vi "Camera Communication.vi"(9 "Modle":string="1", 10 "Trigger Cammand":bool) -> ()   [LabVIEW 2015]
uses:
  Control Button/cameraenum.ctl
  Galobal variable_TI.vi
panel:
  out "error out 2":errorcluster
  out "Boolean":bool
  in  "x":bool
  out "data out 3":string
  out "data out 2":string
  out "error out":errorcluster
  out "data out":string
  # "Meadium=1"
  # "Globle=2"
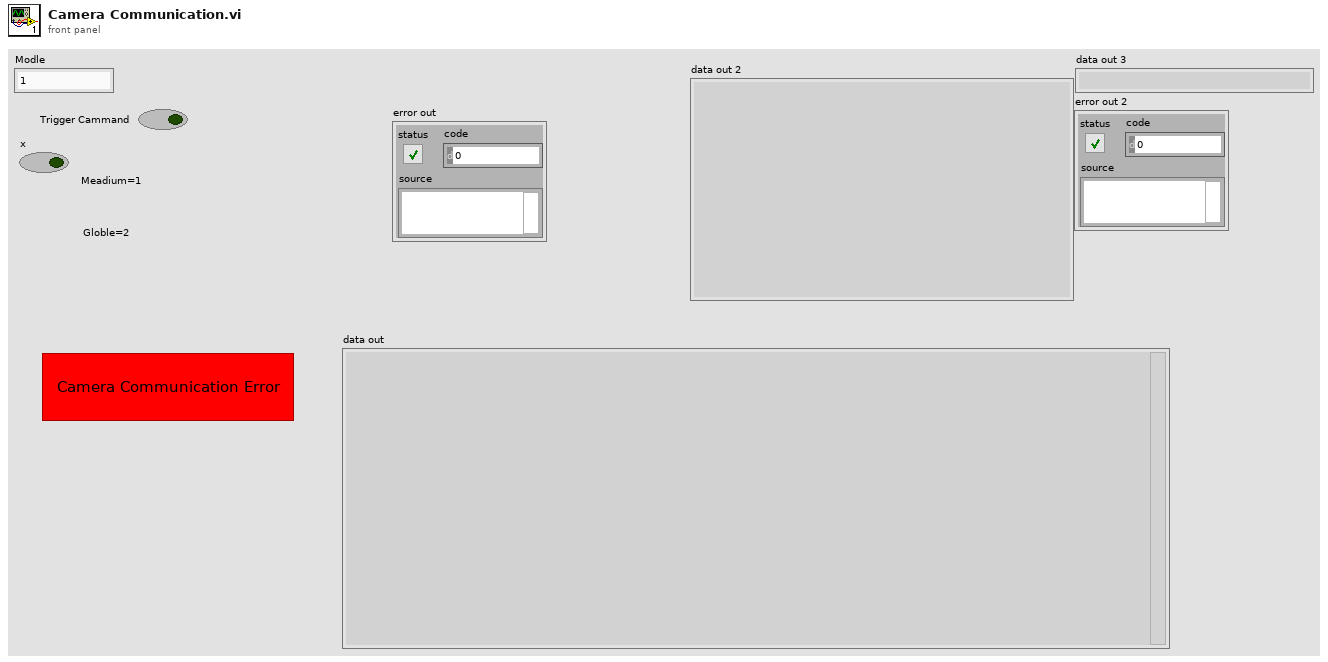
[diagram p1: front panel]
types:
  T1 = enum16{"Standard", "Buffered", "CRLF", "Immediate"}
  T2 = typedef "cameraenum.ctl" = enum16{"Poll event", "Camera Off Mode", "Job Chage", "Camera online  Mode", "Camera trigger Mode", "Read", "Session close"}
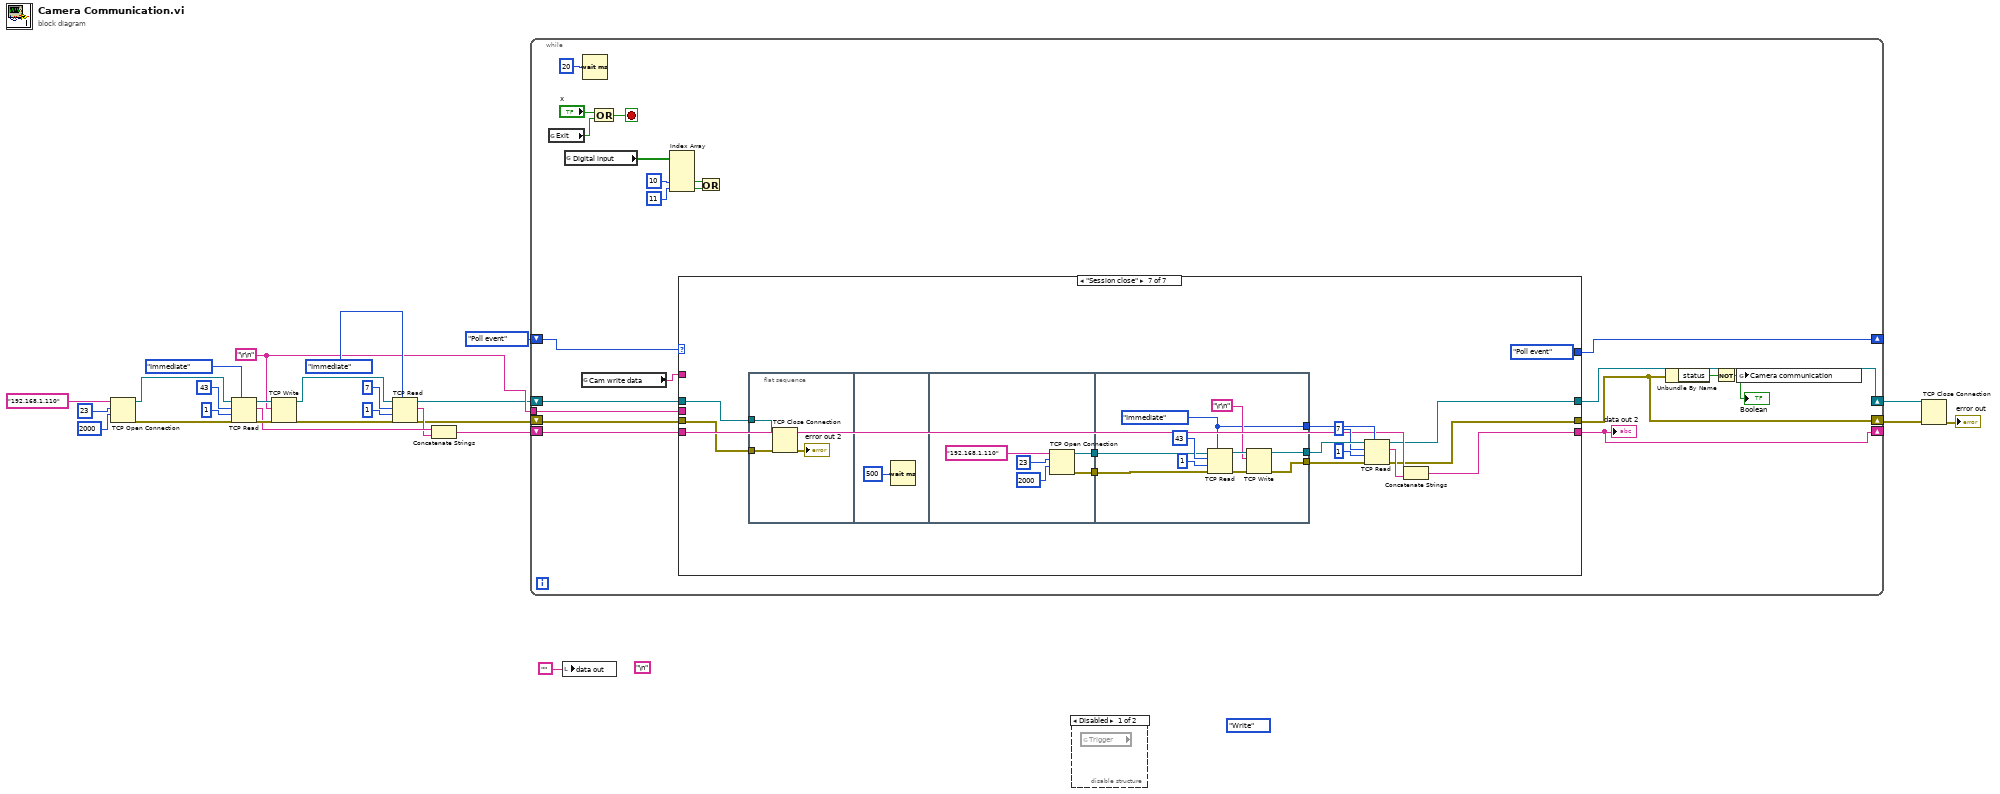
[diagram p0: block diagram]
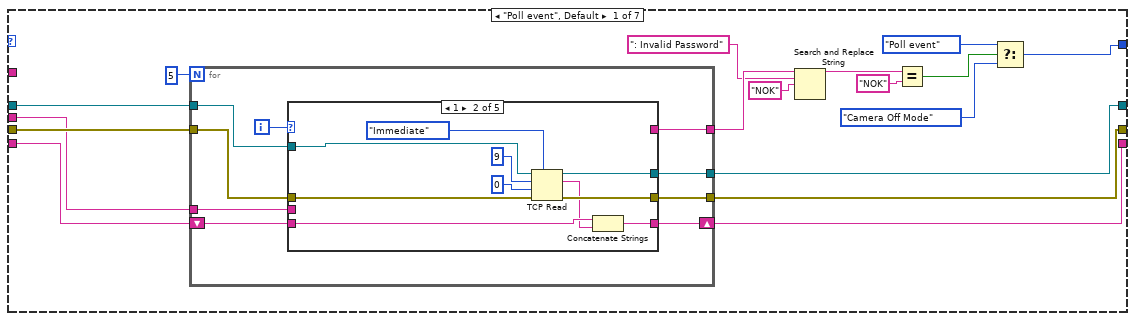
[diagram p3: hidden frame]
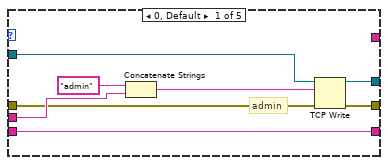
[diagram p4: hidden frame]
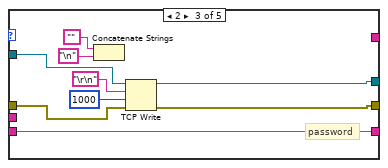
[diagram p5: hidden frame]
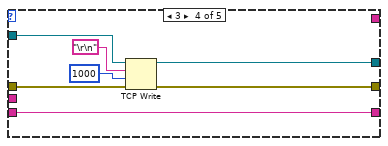
[diagram p6: hidden frame]
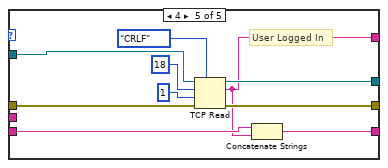
[diagram p7: hidden frame]
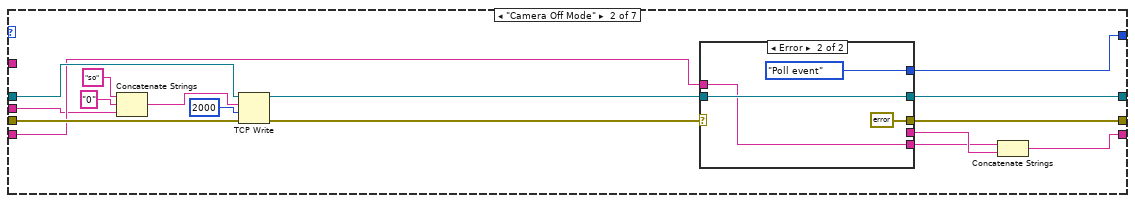
[diagram p8: hidden frame]
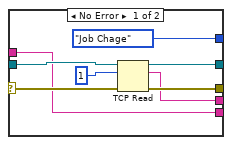
[diagram p9: hidden frame]
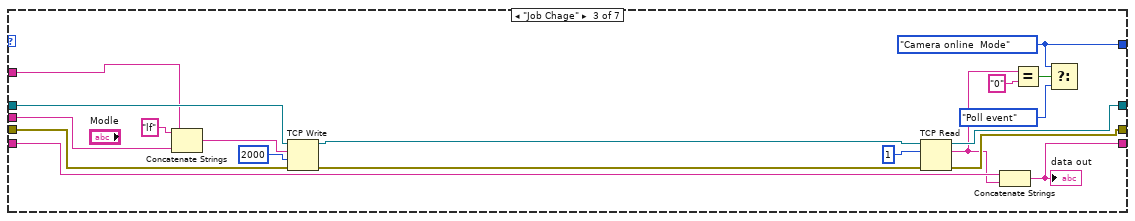
[diagram p10: hidden frame]
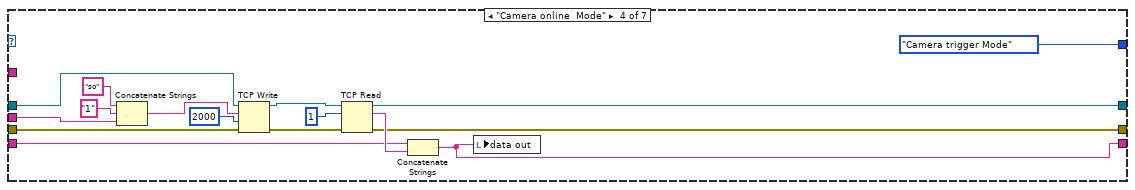
[diagram p11: hidden frame]
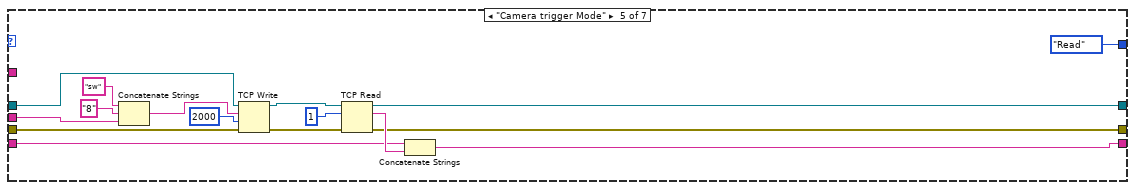
[diagram p12: hidden frame]
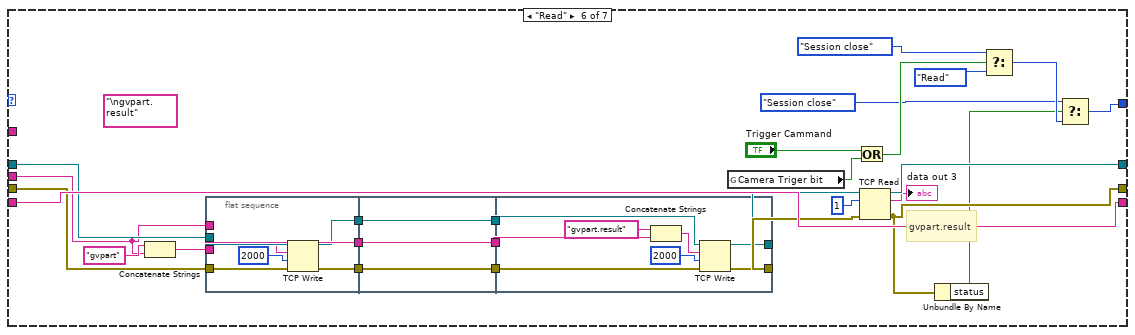
[diagram p13: hidden frame]
diagram:
  (unwired) "\n"
  w4 = "\r\n"
  (unwired) enum16{"Poll event", "Write", "Read", ""}."Write"
  n1 = TCP Open Connection(address="192.168.1.110", remote port or service name=u16 23, timeout ms (60000)=2000) -> (connection ID=w20:refnum<k5>, error out=w19:errorcluster)  [unwired: 2 in]
  n2 = TCP Read(connection ID=w20, bytes to read=43, error in (no error)=w19, 7:T1."Immediate" ("mode (standard)"), 9:1 ("timeout ms (25000)")) -> (connection ID out=w18:refnum<k5>, data out=w15:string, error out=w17:errorcluster)
  n3 = TCP Write(connection ID=w18, data in=w4, error in (no error)=w17) -> (connection ID out=w13:refnum<k5>, error out=w12:errorcluster)  [unwired: 1 in, 1 out]
  n4 = TCP Read(connection ID=w13, bytes to read=7, error in (no error)=w12, 7:T1."Immediate" ("mode (standard)"), 9:1 ("timeout ms (25000)")) -> (connection ID out=w2:refnum<k5>, data out=w14:string, error out=w1:errorcluster)
  n5 = Concatenate Strings(w15, w14) -> (w3:string)
  n6 = while {
    shift-right: [w46] -> _
    shift-left: w3 -> [w45]
    shift-right: [w43] -> _
    shift-left: cameraenum."Poll event" ("Enum") -> [w42]
    shift-right: [w32] -> w6
    shift-left: w2 -> [w47]
    shift-right: [w31] -> w5
    shift-left: w1 -> [w30]
    tunnel: w4 -> [w41]
    stop <- w39 stop-if-true
    n7 = global read "Galobal variable_TI.vi" "Exit"() -> (w40:bool)
    n8 = global read "Galobal variable_TI.vi" "Digital input"() -> (w37:bool[])
    n9 = global read "Galobal variable_TI.vi" "Cam write data"() -> (w27:string)
    n10 = Wait (ms)(milliseconds to wait=u32 20) -> ()  [unwired: 1 out]
    n11 = Compound Arithmetic op=OR("x", w40) -> (w39:bool)
    n12 = Index Array(array=w37, index #3=10 ("index"), index #4=11 ("index")) -> (element #3=w34:bool, element #4=w33:bool)  [unwired: 2 in, 2 out]
    n13 = case shown="\"Session close\"" w42 {
      tunnel: w47 -> [w63 w133 w161 w172 w188 w218 w244]
      tunnel: w30 -> [w62 w132 w160 w171 w187 w216 w243]
      tunnel: [w60 w123 w156 w170 w186 w217 w246] -> w32
      tunnel: [w59 w127 w155 w169 w185 w203 w247] -> w31
      tunnel: [w52 w126 w147 cameraenum."Camera trigger Mode" ("Enum") cameraenum."Read" ("f") w222 cameraenum."Poll event" ("f")] -> w43
      tunnel: [w58 w120 w153 w167 w184 w223 w248] -> w46
      tunnel: w45 -> [w64 w122 w154 w168 w183 w223 w249]
      tunnel: w41 -> [w61 w121 w152 w165 w181 w207 _]
      tunnel: w27 -> [_ _ w146 _ _ _ _]
      frame "Poll event", Default {
        n14 = for {
          N: 5 -> [_]
          tunnel: w61 -> [w72]
          tunnel: w63 -> [w71]
          tunnel: w62 -> [w70]
          tunnel: [w69] -> w60
          tunnel: [w68] -> w59
          shift-right: [w67] -> w58
          shift-left: w64 -> [w66]
          tunnel: [w65] -> w51
          i -> [w73]
          n15 = case shown="1" w73 {
            tunnel: w72 -> [w80 _ _ _ _]
            tunnel: w71 -> [w78 w91 w100 w104 w116]
            tunnel: w70 -> [w77 w90 w99 w103 w108]
            tunnel: [w76 w87 w98 w107 w115] -> w69
            tunnel: [w75 w86 w97 w106 w114] -> w68
            tunnel: [w74 w89 w96 w105 w112] -> w67
            tunnel: w66 -> [w74 w88 w96 w105 w113]
            tunnel: [_ _ _ _ w111] -> w65
            frame 0, Default {
              # "admin"
              n16 = Concatenate Strings("admin", w80) -> (w79:string)
              n17 = TCP Write(connection ID=w78, data in=w79, error in (no error)=w77) -> (connection ID out=w76:refnum<k5>, error out=w75:errorcluster)  [unwired: 1 in, 1 out]
            }
            frame 1 {
              n18 = TCP Read(connection ID=w91, bytes to read=9, error in (no error)=w90, 7:T1."Immediate" ("mode (standard)"), 9:0 ("timeout ms (25000)")) -> (connection ID out=w87:refnum<k5>, data out=w84:string, error out=w86:errorcluster)
              n19 = Concatenate Strings(w88, w84) -> (w89:string)
            }
            frame 2 {
              # "password"
              n20 = Concatenate Strings("", "\n") -> ()  [unwired: 1 out]
              n21 = TCP Write(connection ID=w100, data in="\r\n", error in (no error)=w99, 9:1000 ("timeout ms (25000)")) -> (connection ID out=w98:refnum<k5>, error out=w97:errorcluster)  [unwired: 1 out]
            }
            frame 3 {
              n22 = TCP Write(connection ID=w104, data in="\r\n", error in (no error)=w103, 9:1000 ("timeout ms (25000)")) -> (connection ID out=w107:refnum<k5>, error out=w106:errorcluster)  [unwired: 1 out]
            }
            frame 4 {
              # "User Logged In"
              n23 = TCP Read(connection ID=w116, bytes to read=18, error in (no error)=w108, 7:T1."CRLF" ("mode (standard)"), 9:1 ("timeout ms (25000)")) -> (connection ID out=w115:refnum<k5>, data out=w111:string, error out=w114:errorcluster)
              n24 = Concatenate Strings(w113, w111) -> (w112:string)
            }
          }
        }
        n25 = Search and Replace String(input string=w51, search string=": Invalid Password", replace string="NOK" ("replace string (\"\")")) -> (result string=w48:string)  [unwired: 5 in, 3 out]
        n26 = Equal?(x=w48, y="NOK") -> (x = y?=w55:bool)
        n27 = Select(t=cameraenum."Poll event" ("Enum"), s=w55, f=cameraenum."Camera Off Mode") -> (s? t:f=w52:T2)
      }
      frame "Camera Off Mode" {
        n28 = Concatenate Strings("so" ("data in"), "0" ("string"), w121) -> (w129:string)
        n29 = TCP Write(connection ID=w133, data in=w129, error in (no error)=w132, 9:2000 ("timeout ms (25000)")) -> (connection ID out=w124:refnum<k5>, error out=w128:errorcluster)  [unwired: 1 out]
        n30 = case shown="Error" w128 {
          selector: w128 -> [w137 _]
          tunnel: [w136 errorcluster {"status"=FALSE, "code"=0, "source"=""} ("error IO")] -> w127
          tunnel: [cameraenum."Job Chage" ("Enum") cameraenum."Poll event" ("Enum")] -> w126
          tunnel: w124 -> [w139 w143]
          tunnel: [w138 w143] -> w123
          tunnel: w122 -> [w135 w142]
          tunnel: [w135 w142] -> w118
          tunnel: [w134 _] -> w119
          frame No Error {
            n31 = TCP Read(connection ID=w139, bytes to read=1, error in (no error)=w137) -> (connection ID out=w138:refnum<k5>, data out=w134:string, error out=w136:errorcluster)  [unwired: 2 in]
          }
          frame Error {
          }
        }
        n32 = Concatenate Strings(w118, w119) -> (w120:string)
      }
      frame "Job Chage" {
        w147 = cameraenum."Camera online  Mode" ("Enum")
        n33 = Concatenate Strings("lf" ("data in"), w146, w152) -> (w163:string)
        n34 = TCP Write(connection ID=w161, data in=w163, error in (no error)=w160, 9:2000 ("timeout ms (25000)")) -> (connection ID out=w157:refnum<k5>, error out=w159:errorcluster)  [unwired: 1 out]
        n35 = TCP Read(connection ID=w157, bytes to read=1, error in (no error)=w159) -> (connection ID out=w156:refnum<k5>, data out=w151:string, error out=w155:errorcluster)  [unwired: 2 in]
        n36 = Concatenate Strings(w154, w151) -> (w153:string)
        "data out" <- w153
        n37 = Equal?(x=w151, y="0") -> (x = y?=w149:bool)
        n38 = Select(t=w147, s=w149, f=cameraenum."Poll event" ("Enum")) -> ()  [unwired: 1 out]
      }
      frame "Camera online  Mode" {
        n39 = Concatenate Strings("so" ("data in"), "1" ("string"), w165) -> (w178:string)
        n40 = TCP Write(connection ID=w172, data in=w178, error in (no error)=w171, 9:2000 ("timeout ms (25000)")) -> (connection ID out=w174:refnum<k5>, error out=w176:errorcluster)  [unwired: 1 out]
        n41 = TCP Read(connection ID=w174, bytes to read=1, error in (no error)=w176) -> (connection ID out=w170:refnum<k5>, data out=w173:string, error out=w169:errorcluster)  [unwired: 2 in]
        n42 = Concatenate Strings(w168, w173) -> (w167:string)
        n43 = local write "data out"(w167) -> ()
      }
      frame "Camera trigger Mode" {
        n44 = Concatenate Strings("sw" ("data in"), "8" ("string"), w181) -> (w194:string)
        n45 = TCP Write(connection ID=w188, data in=w194, error in (no error)=w187, 9:2000 ("timeout ms (25000)")) -> (connection ID out=w190:refnum<k5>, error out=w192:errorcluster)  [unwired: 1 out]
        n46 = TCP Read(connection ID=w190, bytes to read=1, error in (no error)=w192) -> (connection ID out=w186:refnum<k5>, data out=w189:string, error out=w185:errorcluster)  [unwired: 2 in]
        n47 = Concatenate Strings(w183, w189) -> (w184:string)
      }
      frame "Read" {
        (unwired) "\ngvpart.result" ("data in")
        # "gvpart.result"
        n48 = Concatenate Strings("gvpart" ("data in"), w207) -> (w206:string)
        n49 = flat-sequence {
          tunnel: w207 -> [w230]
          tunnel: w216 -> [w228]
          tunnel: w218 -> [w227]
          tunnel: [w226] -> w211
          tunnel: [w225] -> w210
          tunnel: [w230] -> w209
          tunnel: w206 -> [w224]
          tunnel: [w233] -> w214
          tunnel: [w232] -> w213
          tunnel: [w231] -> w212
          tunnel: w211 -> [w233]
          tunnel: w210 -> [w232]
          tunnel: w209 -> [w231]
          tunnel: [w239] -> w221
          tunnel: [w238] -> w219
          tunnel: w214 -> [w237]
          tunnel: w213 -> [w236]
          tunnel: w212 -> [w234]
          frame #0 {
            n50 = TCP Write(connection ID=w227, data in=w224, error in (no error)=w228, 9:2000 ("timeout ms (25000)")) -> (connection ID out=w226:refnum<k5>, error out=w225:errorcluster)  [unwired: 1 out]
          }
          frame #1 {
          }
          frame #2 {
            n51 = Concatenate Strings("gvpart.result" ("data in"), w234) -> (w241:string)
            n52 = TCP Write(connection ID=w237, data in=w241, error in (no error)=w236, 9:2000 ("timeout ms (25000)")) -> (connection ID out=w238:refnum<k5>, error out=w239:errorcluster)  [unwired: 1 out]
          }
        }
        n53 = global read "Galobal variable_TI.vi" "Camera Triger bit"() -> (w205:bool)
        n54 = Or(x="Trigger Cammand", y=w205) -> (x .or. y?=w200:bool)
        n55 = TCP Read(connection ID=w219, bytes to read=1, error in (no error)=w221) -> (connection ID out=w217:refnum<k5>, data out=→"data out 3":string, error out=w203:errorcluster)  [unwired: 2 in]
        n56 = Unbundle By Name(w203) -> ("status"=w198:bool)
        n57 = Select(t=cameraenum."Session close", s=w200, f=cameraenum."Read") -> (s? t:f=w199:T2)
        n58 = Select(t=cameraenum."Session close", s=w198, f=w199) -> (s? t:f=w222:T2)
      }
      frame "Session close" {
        n59 = flat-sequence {
          tunnel: w244 -> [w258]
          tunnel: w243 -> [w257]
          tunnel: [w262] -> w256
          tunnel: [w261] -> w242
          tunnel: w256 -> [w270]
          tunnel: [w269] -> w253
          tunnel: [w268] -> w254
          tunnel: [w267] -> w255
          tunnel: w242 -> [w266]
          frame #0 {
            n60 = TCP Close Connection(connection ID=w258, error in (no error)=w257) -> (error out=→"error out 2":errorcluster)  [unwired: 1 in, 1 out]
          }
          frame #1 {
            n61 = Wait (ms)(milliseconds to wait=u32 500) -> ()  [unwired: 1 out]
          }
          frame #2 {
            n62 = TCP Open Connection(address="192.168.1.110", remote port or service name=u16 23, timeout ms (60000)=2000) -> (connection ID=w261:refnum<k5>, error out=w262:errorcluster)  [unwired: 2 in]
          }
          frame #3 {
            w267 = T1."Immediate" ("mode (standard)")
            n63 = TCP Read(connection ID=w266, bytes to read=43, error in (no error)=w270, 7:w267, 9:1 ("timeout ms (25000)")) -> (connection ID out=w274:refnum<k5>, error out=w273:errorcluster)  [unwired: 1 out]
            n64 = TCP Write(connection ID=w274, data in="\r\n", error in (no error)=w273) -> (connection ID out=w269:refnum<k5>, error out=w268:errorcluster)  [unwired: 1 in, 1 out]
          }
        }
        n65 = TCP Read(connection ID=w253, bytes to read=7, error in (no error)=w254, 7:w255, 9:1 ("timeout ms (25000)")) -> (connection ID out=w246:refnum<k5>, data out=w251:string, error out=w247:errorcluster)
        n66 = Concatenate Strings(w249, w251) -> (w248:string)
      }
    }
    "data out 2" <- w46
    n67 = Or(x=w34, y=w33) -> ()  [unwired: 1 out]
    n68 = Unbundle By Name(w31) -> ("status"=w29:bool)
    n69 = Not(x=w29) -> (.not. x?=w28:bool)
    "Boolean" <- w28
    n70 = global write "Galobal variable_TI.vi" "Camera communication"(w28) -> ()
  }
  n71 = local write "data out"("") -> ()
  n72 = disable-structure shown="Disabled" {
    frame Disabled {
      n73 = global read "Galobal variable_TI.vi" "Trigger"() -> ()  [unwired: 1 out]
    }
    frame Enabled {
    }
  }
  n74 = TCP Close Connection(connection ID=w6, error in (no error)=w5) -> (error out=→"error out":errorcluster)  [unwired: 1 in, 1 out]
